vi "Post-Build Action.vi"(5 "Files Generated by Build":path[](array[path]), 6 "Top Level/Always Included VIs":path[](array[path]), 7 "Destination Path":path, 8 "error in (no error)":errorcluster, 9 "Target Name":string, 10 "Build Specification Name":string, 11 "Project Path":path) -> (0 "error out":errorcluster)   [LabVIEW 2020, in "ni-veristand-steps-runtime-lib.lvlib"]
uses:
  ni-veristand-steps-runtime-lib.lvlib
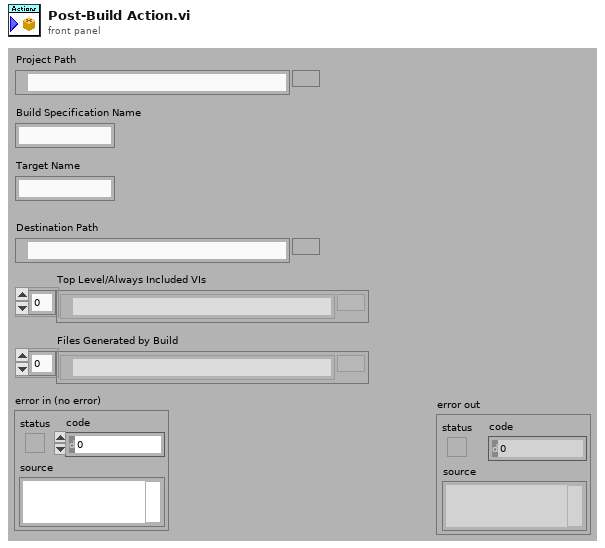
[diagram p1: front panel]
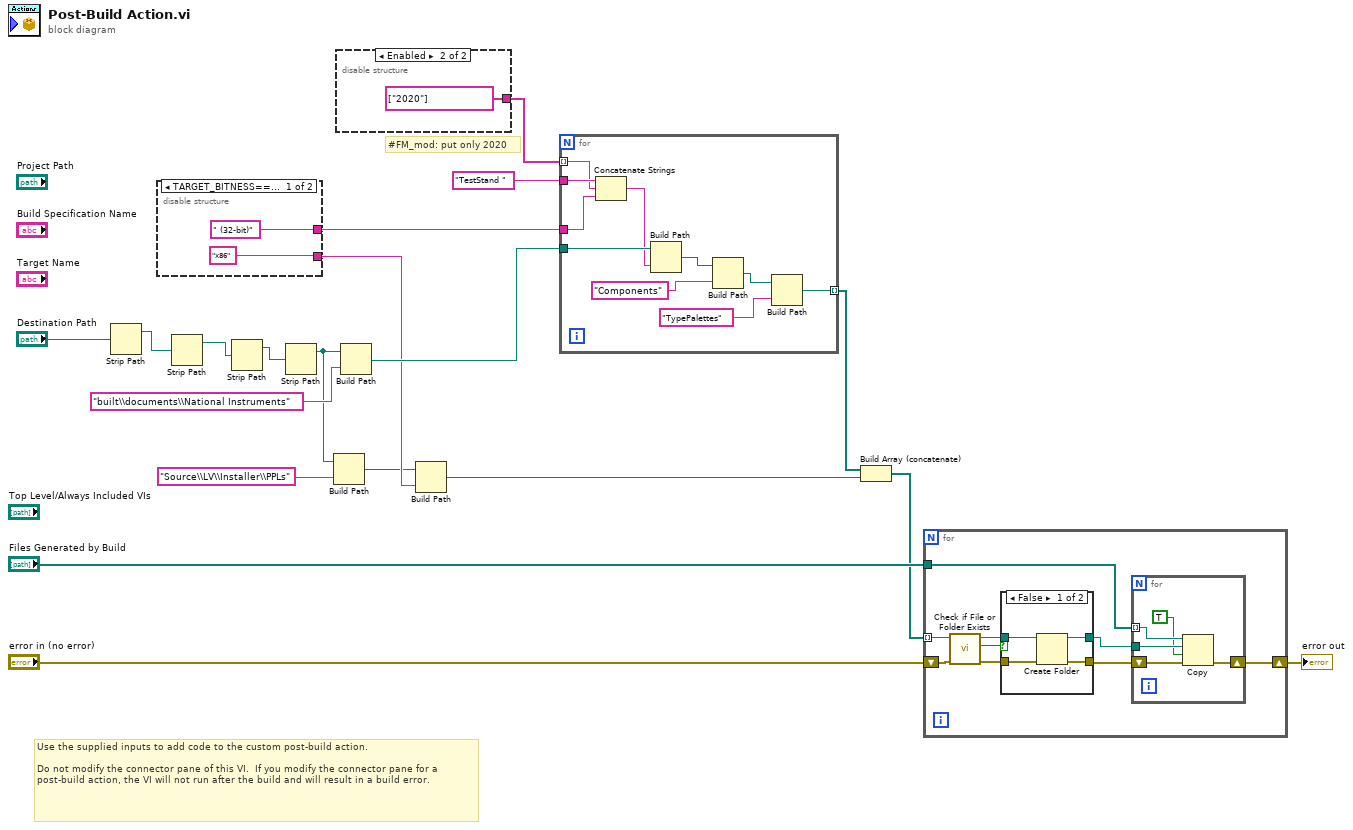
[diagram p0: block diagram]
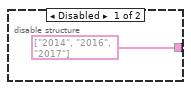
[diagram p2: hidden frame]
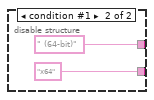
[diagram p4: hidden frame]
diagram:
  # "#FM_mod: put only 2020"
  # "Use the supplied inputs to add code to the custom post-build action.\n\nDo not modify the connector pane of this VI.  If you modify the connector pane for a post-build action, the VI will not run after the build and will result in a build error."
  n1 = Strip Path(path="Destination Path") -> (stripped path=w15:path)  [unwired: 1 out]
  n2 = disable-structure shown="TARGET_BITNESS==32, Default" {
    disable-tunnel: [" (32-bit)" " (64-bit)"] -> w9
    disable-tunnel: ["x86" "x64"] -> w5
    frame condition #0 (active) {
    }
    frame condition #1 {
    }
  }
  n3 = Strip Path(path=w15) -> (stripped path=w14:path)  [unwired: 1 out]
  n4 = Strip Path(path=w14) -> (stripped path=w13:path)  [unwired: 1 out]
  n5 = Strip Path(path=w13) -> (stripped path=w7:path)  [unwired: 1 out]
  n6 = Build Path(base path=w7, name or relative path="Source\\LV\\Installer\\PPLs") -> (appended path=w4:path)
  n7 = disable-structure shown="Enabled" {
    disable-tunnel: [string[] ["2014", "2016", "2017"] string[] ["2020"]] -> w10
    frame Disabled {
    }
    frame Enabled {
    }
  }
  n8 = Build Path(base path=w7, name or relative path="built\\documents\\National Instruments") -> (appended path=w8:path)
  n9 = Build Path(base path=w4, name or relative path=w5) -> (appended path=w2:path)
  n10 = for {
    tunnel: "TestStand " ("string") -> [w35]
    tunnel: w10 -> [w34] mode=indexing
    tunnel: w9 -> [w33]
    tunnel: w8 -> [w32]
    tunnel: [w26] -> w3 mode=indexing
    n11 = Concatenate Strings(w35, w34, w33) -> (w31:string)
    n12 = Build Path(base path=w32, name or relative path=w31) -> (appended path=w30:path)
    n13 = Build Path(base path=w30, name or relative path="Components") -> (appended path=w28:path)
    n14 = Build Path(base path=w28, name or relative path="TypePalettes") -> (appended path=w26:path)
  }
  n15 = Build Array (concatenate)(w3, w2) -> (w1:path[])
  n16 = for {
    tunnel: "Files Generated by Build" -> [w37]
    shift-right: [w39] -> w18
    shift-left: "error in (no error)" -> [w44]
    tunnel: w1 -> [w36] mode=indexing
    n17 = call <vilib>:"Check if File or Folder Exists.vi"("error in (no error)"=w44, "path"=w36) -> ("error out"=w43:errorcluster, "file or folder exists?"=w42:bool, "dup path"=w41:path)  [unwired: 7 in]
    n18 = case shown="False" w42 {
      tunnel: w43 -> [w53 w54]
      tunnel: w41 -> [w51 w55]
      tunnel: [w52 w54] -> w40
      tunnel: [w50 w55] -> w38
      frame False {
        n19 = Create Folder(path (use dialog)=w51, error in=w53) -> (created path=w50:path, error out=w52:errorcluster)  [unwired: 1 in, 1 out]
      }
      frame True {
      }
    }
    n20 = for {
      tunnel: w38 -> [w47]
      shift-right: [w48] -> w39
      shift-left: w40 -> [w49]
      tunnel: w37 -> [w46] mode=indexing
      n21 = Copy(8:w49, 9:TRUE ("overwrite (F)"), 10:w47, 11:w46) -> (0:w48:errorcluster)  [unwired: 1 in, 2 out]
    }
  }
  "error out" <- w18
